vi "Append String to StdOut.vi"(4 "error in (no error)":errorcluster, 7 "text":string) -> (0 "error out":errorcluster)   [LabVIEW 2015, in "StdOut Operations.lvlib"]
uses:
  StdOut Operations.lvlib
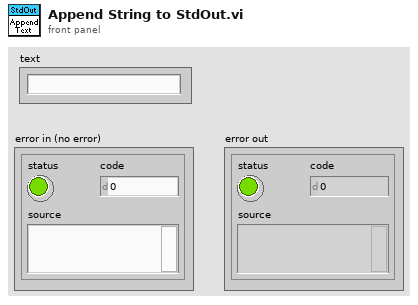
[diagram p1: front panel]
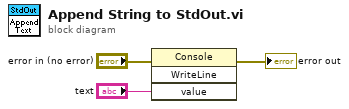
[diagram p0: block diagram]
diagram:
  n1 = invoke class="Console" method="WriteLine"(error in="error in (no error)", "value"="text") -> (error out=→"error out":errorcluster)  [unwired: 2 in, 3 out]
